vi "Address Generator.vi"(6 "Reset":bool, 8 "Input Valid":bool, 10 "Input Data Valid Array":bool[](array[boolean])=[FALSE, FALSE], 11 "Input Data":fxp<+/-,16,2>[](array[numeric])=[0.0, 0.0]) -> (0 "Output Valid":bool, 2 "Data 2":T1, 3 "Data 1":T2, 4 "Address 1":i16, 5 "Address 0":i16)   [LabVIEW 2012]
uses:
  <vilib>/rvi/FXPMathLib/basic elements/FxpDiscreteDelay/XNode/nifxpmath_DiscreteDelay.xnode
  <vilib>/rvi/FXPMathLib/FxpInterpret/XNode/nifxpmath_Interpret.xnode
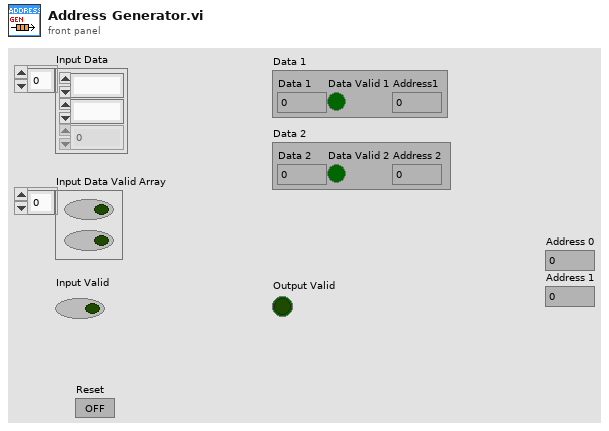
[diagram p1: front panel]
types:
  T1 = cluster{"Data 2":u16, "Data Valid 2":bool, "Address 2":u16}
  T2 = cluster{"Data 1":u16, "Data Valid 1":bool, "Address1":u16}
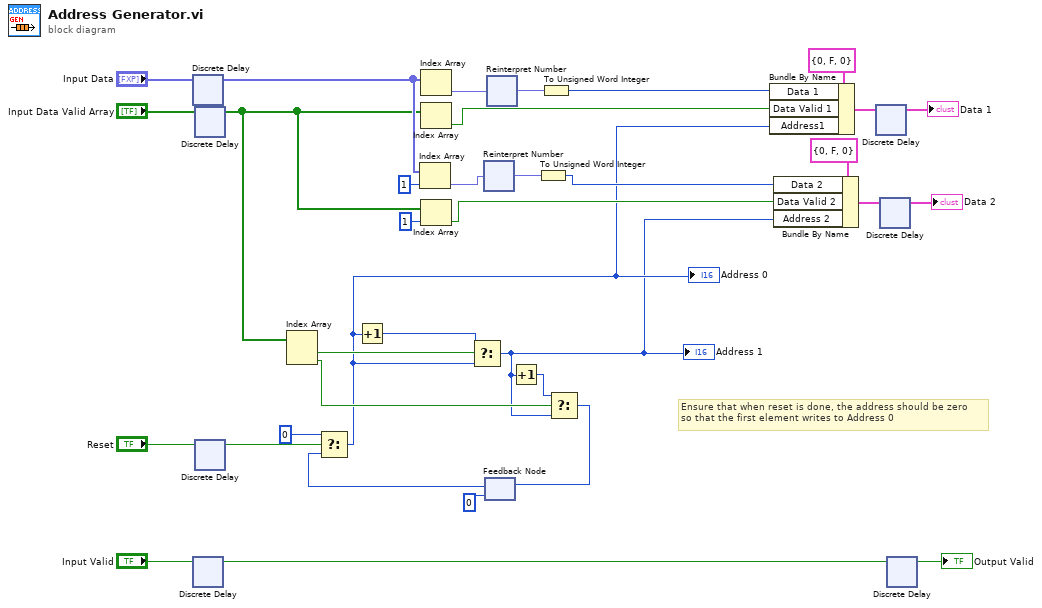
[diagram p0: block diagram]
diagram:
  # "Ensure that when reset is done, the address should be zero\nso that the first element writes to Address 0"
  n1 = xnode "Discrete Delay"("D"="Input Data") -> ("Q"=w10:fxp<+/-,16,2>[])
  n2 = xnode "Discrete Delay"("D"="Input Valid") -> ("Q"=w7:bool)
  n3 = xnode "Discrete Delay"("D"="Input Data Valid Array") -> ("Q"=w9:bool[])
  n4 = xnode "Discrete Delay"("D"="Reset") -> ("Q"=w8:bool)
  n5 = Index Array(array=w9) -> (element #1=w33:bool, element #2=w32:bool)  [unwired: 2 in]
  n6 = Index Array(array=w10, index=1) -> (element=w15:fxp<+/-,16,2>)
  n7 = Index Array(array=w10) -> (element=w19:fxp<+/-,16,2>)  [unwired: 1 in]
  n8 = Index Array(array=w9) -> (element=w27:bool)  [unwired: 1 in]
  n9 = Index Array(array=w9, index=1) -> (element=w23:bool)
  n10 = xnode "Reinterpret Number"("x"=w15) -> ("y"=w16:fxp<+,16,16>)
  n11 = feedback #1(i16 0) -> (w29:i16)
  n12 = Select(t=i16 0, s=w8, f=w29) -> (s? t:f=w3:i16)
  "Address 0" <- w3
  n13 = Increment(x=w3) -> (x+1=w34:i16)
  n14 = Select(t=w34, s=w33, f=w3) -> (s? t:f=w1:i16)
  "Address 1" <- w1
  n15 = xnode "Reinterpret Number"("x"=w19) -> ("y"=w18:fxp<+,16,16>)
  n16 = Increment(x=w1) -> (x+1=w2:i16)
  n17 = To Unsigned Word Integer(number=w16) -> (unsigned 16bit integer=w14:u16)
  n18 = To Unsigned Word Integer(number=w18) -> (unsigned 16bit integer=w17:u16)
  n19 = Select(t=w2, s=w32, f=w1) -> (s? t:f=w22:i16)
  n20 = feedback-in #1(w22) -> ()
  n21 = Bundle By Name(cluster=T2 {"Data 1"=0, "Data Valid 1"=FALSE, "Address1"=0} ("Bank0 Data"), "Data 1"=w17, "Data Valid 1"=w27, "Address1"=w3) -> (w13:T2)
  n22 = Bundle By Name(cluster=T1 {"Data 2"=0, "Data Valid 2"=FALSE, "Address 2"=0} ("Bank1 Data"), "Data 2"=w14, "Data Valid 2"=w23, "Address 2"=w1) -> (w12:T1)
  n23 = xnode "Discrete Delay"("D"=w13) -> ("Q"=→"Data 1":T2)
  n24 = xnode "Discrete Delay"("D"=w12) -> ("Q"=→"Data 2":T1)
  n25 = xnode "Discrete Delay"("D"=w7) -> ("Q"=→"Output Valid":bool)
